vi "Color to .net argb.vi"(8 "error in (no error)":errorcluster, 11 "Color":cluster{"Color":u32, "Alpha":u8}) -> (0 "error out":errorcluster, 3 "FromArgb":refnum<k24>)   [LabVIEW 2020, in "Glyph .NET.lvlib" / "Drawer .Net.lvclass"]
uses:
  Drawer .Net.lvclass
  System.Drawing
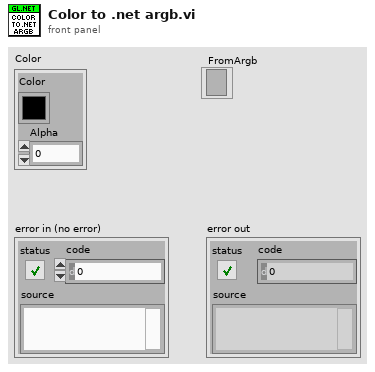
[diagram p1: front panel]
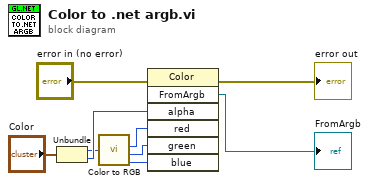
[diagram p0: block diagram]
diagram:
  n1 = Unbundle("Color") -> ("Color"=w8:u32, "Alpha"=w9:u8)
  n2 = call <vilib>:"Color to RGB.vi"("Color"=w8) -> ("R"=w7:u8, "G"=w6:u8, "B"=w5:u8)  [unwired: 1 out]
  n3 = invoke class="Color" method="FromArgb"(error in="error in (no error)", "alpha"=w9, "red"=w7, "green"=w6, "blue"=w5) -> (error out=→"error out":errorcluster, "FromArgb"=→"FromArgb":refnum<k24>)  [unwired: 2 in, 5 out]
